vi "Web_Client.vi"(0 "Channel Name":string="Froude:NPL:Atmos_Press") -> (1 "Value":dbl format="%.2f", 2 "Time Of Value (s)":dbl format="%.2f")   [LabVIEW 2015]
uses:
  ADAM Client/Sub VIs/ADAM Controls/Remember_value_mode.ctl
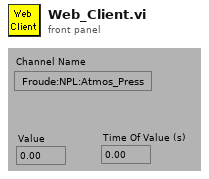
[diagram p1: front panel]
types:
  T1 = typedef "Remember_value_mode.ctl" = enum16{"Read only", "Read and Write"}
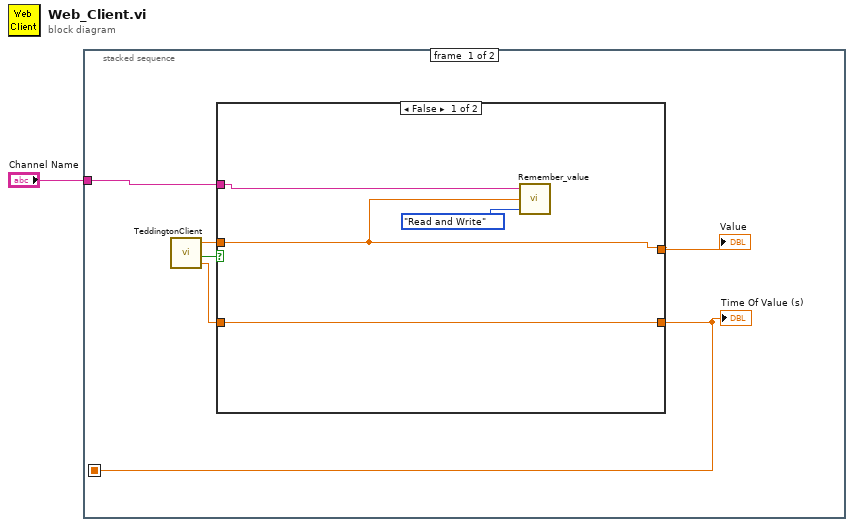
[diagram p0: block diagram]
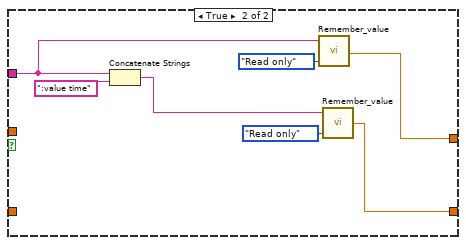
[diagram p2: hidden frame]
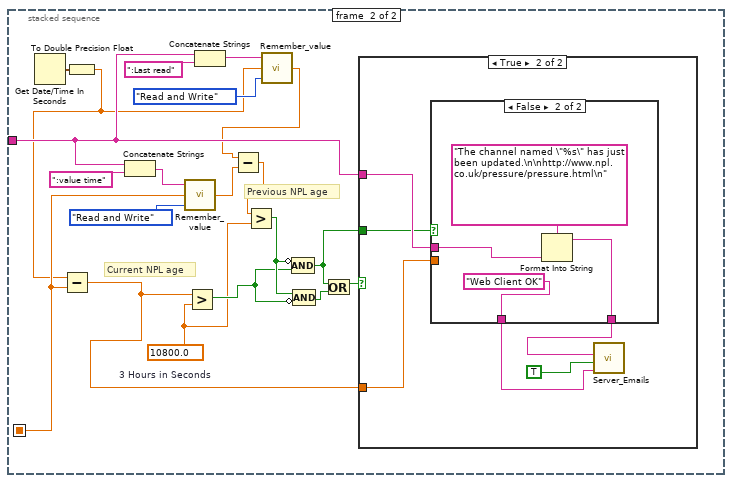
[diagram p3: hidden frame]
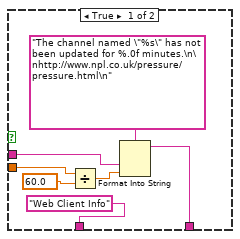
[diagram p5: hidden frame]
diagram:
  n1 = stacked-sequence {
    seq-local: [w6 _] -> [_ w26]
    tunnel: "Channel Name" -> [w5 w21]
    frame #0 {
      n2 = call "TeddingtonClient.vi"() -> ("Time Of Value (s)"=w2:dbl, "Error"=w4:bool, "Sea level Pressure String/mBar"=w3:dbl)
      n3 = case shown="False" w4 {
        tunnel: [w8 w12] -> w7
        tunnel: [w11 w13] -> w6
        tunnel: w5 -> [w9 w15]
        tunnel: w3 -> [w8 _]
        tunnel: w2 -> [w11 _]
        frame False {
          n4 = call "Remember_value.vi"("Mode"=Remember_value_mode."Read and Write", "Input Value"=w8, "Ch name"=w9) -> ()  [unwired: 1 out]
        }
        frame True {
          n5 = Concatenate Strings(w15, ":value time" ("Substring")) -> (w14:string)
          n6 = call "Remember_value.vi"("Mode"=Remember_value_mode."Read only", "Ch name"=w15) -> ("Output Value"=w12:dbl)  [unwired: 1 in]
          n7 = call "Remember_value.vi"("Mode"=Remember_value_mode."Read only", "Ch name"=w14) -> ("Output Value"=w13:dbl)  [unwired: 1 in]
        }
      }
      "Time Of Value (s)" <- w6
      "Value" <- w7
    }
    frame #1 {
      w30 = 10800.0  # 3 Hours in Seconds
      # "Previous NPL age"
      # "Current NPL age"
      n8 = Get Date/Time In Seconds() -> (seconds since 1Jan1904=w29:timestamp)
      n9 = To Double Precision Float(number=w29) -> (double precision float=w20:dbl)
      n10 = Subtract(x=w20, y=w26) -> (x-y=w25:dbl)
      n11 = Concatenate Strings(w21, ":value time" ("Substring")) -> (w36:string)
      n12 = call "Remember_value.vi"("Mode"=Remember_value_mode."Read and Write", "Input Value"=w26, "Ch name"=w36) -> ("Output Value"=w28:dbl)
      n13 = Greater?(x=w25, y=w30) -> (0:w34:bool)
      n14 = Concatenate Strings(w21, ":Last read" ("Substring")) -> (w22:string)
      n15 = call "Remember_value.vi"("Mode"=Remember_value_mode."Read and Write", "Input Value"=w20, "Ch name"=w22) -> ("Output Value"=w19:dbl)
      n16 = Subtract(x=w19, y=w28) -> (x-y=w27:dbl)
      n17 = Greater?(x=w27, y=w30) -> (0:w35:bool)
      n18 = Compound Arithmetic op=AND(invert w35, w34) -> (w31:bool)
      n19 = Compound Arithmetic op=AND(w35, invert w34) -> (w33:bool)
      n20 = Or(x=w31, y=w33) -> (x .or. y?=w32:bool)
      n21 = case shown="True" w32 {
        tunnel: w25 -> [_ w44]
        tunnel: w21 -> [_ w43]
        tunnel: w31 -> [_ w41]
        frame False {
        }
        frame True {
          n22 = case shown="False" w41 {
            tunnel: w44 -> [w49 _]
            tunnel: w43 -> [w51 w55]
            tunnel: [w46 w53] -> w42
            tunnel: ["Web Client Info" ("Subject") "Web Client OK" ("Subject")] -> w39
            frame True {
              n23 = Divide(x=w49, y=60.0) -> (x/y=w48:dbl)
              n24 = Format Into String(format string="The channel named \"%s\" has not been updated for %.0f minutes.\n\nhttp://www.npl.co.uk/pressure/pressure.html\n" ("Format String"), w51, w48) -> (resulting string=w46:string)  [unwired: 2 in, 1 out]
            }
            frame False {
              n25 = Format Into String(format string="The channel named \"%s\" has just been updated.\n\nhttp://www.npl.co.uk/pressure/pressure.html\n" ("Format String"), w55) -> (resulting string=w53:string)  [unwired: 2 in, 1 out]
            }
          }
          n26 = call "Server_Emails.vi"("Message"=w42, "Contact All clients?"=TRUE, "Subject"=w39) -> ()  [unwired: 2 in, 3 out]
        }
      }
    }
  }
